vi "updateScrnSep.vi"() -> ()   [LabVIEW 2015]
panel:
  in  "btnScrnSets":bool caption="Update Screen Sets"
  in  "screenSet_2":sgl=1.0 caption="Inner" format="%.2f"
  in  "screenSet_1":sgl=1.0 caption="Outer" format="%.2f"
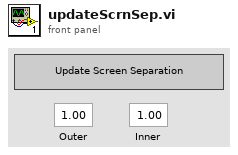
[diagram p1: front panel]
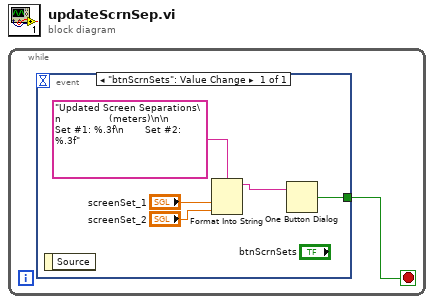
[diagram p0: block diagram]
diagram:
  n1 = while {
    stop <- w1 stop-if-true
    n2 = event shown="[0] \"btnScrnSets\": Value Change" {
      selector: _ -> [_]
      dyn-events: _ -> [_]
      timeout: _ -> [_]
      tunnel: [w2] -> w1
      event "btnScrnSets": Value Change {
        n3 = event-data() -> ()  [unwired: 1 in, 1 out]
        n4 = Format Into String(format string="Updated Screen Separations\n                (meters)\n\n       Set #1: %.3f\n       Set #2: %.3f", "screenSet_1", "screenSet_2") -> (resulting string=w6:string)  [unwired: 2 in, 1 out]
        n5 = One Button Dialog(message=w6) -> (true=w2:bool)  [unwired: 1 in]
      }
    }
  }
